vi "DisconnectCameraRslt.vi"(8 "error in (no error)":errorcluster, 11 "CameraTestingENI":refnum<class "CameraTestingENI.lvclass">) -> (0 "error out":errorcluster, 3 "CameraTestingENI":refnum<class "CameraTestingENI.lvclass">)   [LabVIEW 2020, in "CameraTestingProxy.lvlib" / "CameraTestingENI.lvclass"]
uses:
  CameraTestingENI.lvclass
  CameraTestingENI.lvclass/CameraTestingENI.ctl
  72763862-d66b-47c7-8229-399c68cb3088.vi
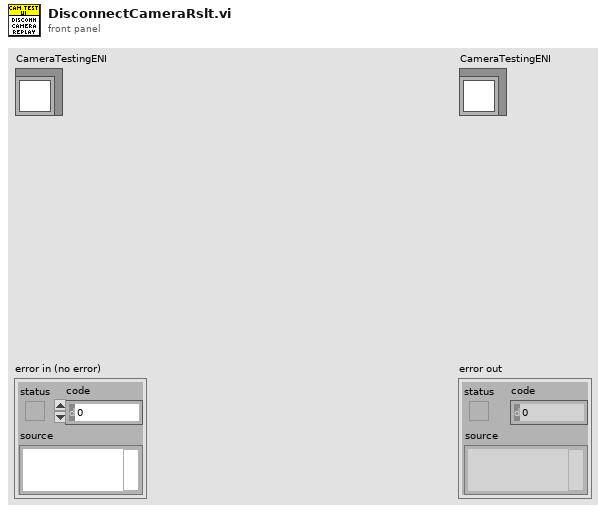
[diagram p1: front panel]
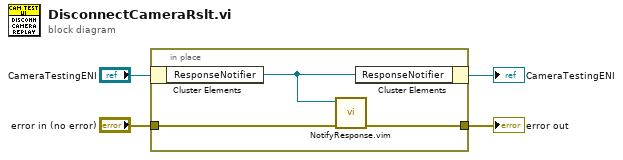
[diagram p0: block diagram]
diagram:
  n1 = in-place {
    in-place-border: "error in (no error)" -> [w6]
    in-place-border: [w7] -> w1
    n2 = in-place-cluster #1("CameraTestingENI") -> ("ResponseNotifier"=w5:refnum<notifier>)
    n3 = call "NotifyResponse.vim"("error in (no error)"=w6, "ResponseNotifier"=w5) -> ("error out"=w7:errorcluster)  [unwired: 9 in]
    n4 = in-place-cluster #1("ResponseNotifier"=w5) -> (→"CameraTestingENI":refnum<class "CameraTestingENI.lvclass">)
  }
  "error out" <- w1
